vi "mean_point_distance.vi"(2 "Pointset 1":cluster{"X":dbl, "Y":dbl}[](array[cluster]), 3 "Pointset 2":cluster{"X":dbl, "Y":dbl}[](array[cluster])) -> (0 "standard deviation":dbl format="%0.2f", 1 "mean distance":dbl format="%0.2f")   [LabVIEW 2019]
uses:
  <vilib>/Analysis/NI_AALBase.lvlib
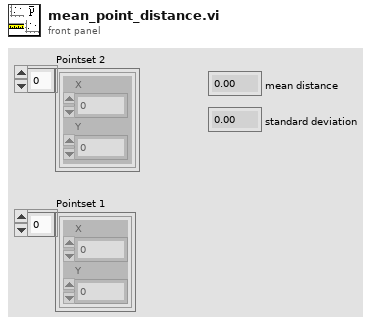
[diagram p1: front panel]
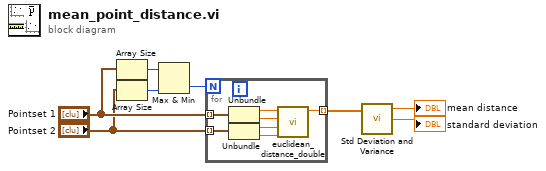
[diagram p0: block diagram]
diagram:
  n1 = Array Size(array="Pointset 1") -> (size(s)=w6:i32)
  n2 = Array Size(array="Pointset 2") -> (size(s)=w5:i32)
  n3 = Max & Min(x=w6, y=w5) -> (min(x,y)=w4:i32)  [unwired: 1 out]
  n4 = for {
    N: w4 -> [_]
    tunnel: "Pointset 2" -> [w14] mode=indexing
    tunnel: "Pointset 1" -> [w15] mode=indexing
    tunnel: [w9] -> w3 mode=indexing
    n5 = Unbundle(w15) -> ("X"=w13:dbl, "Y"=w12:dbl)
    n6 = Unbundle(w14) -> ("X"=w11:dbl, "Y"=w10:dbl)
    n7 = call "euclidean_distance_double.vi"("Point 2 Y"=w10, "Point 2 X"=w11, "Point 1 Y"=w12, "Point 1 X"=w13) -> ("Distance"=w9:dbl)  [unwired: 7 in]
  }
  n8 = call <vilib>:"Std Deviation and Variance.vi"("X"=w3) -> ("mean"=→"mean distance":dbl, "standard deviation"=→"standard deviation":dbl)  [unwired: 1 in, 1 out]
